vi "Test.MATLAB.vi"() -> ()   [LabVIEW 2014]
panel:
  out "Now (us)":dbl=1.0 format="%.2f"
  in  "Parameter":u16(ring) items=["Frequency (MHz)", "Amplitude (dBm)", "Phase (Pi)"]
  in  "Start":dbl=1.0 format="%.3f"
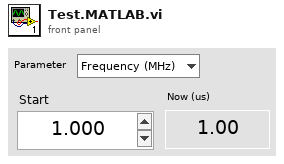
[diagram p1: front panel]
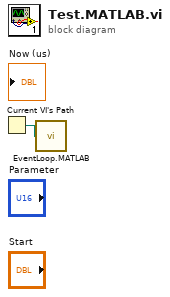
[diagram p0: block diagram]
diagram:
  n1 = Current VI's Path() -> (path=w1:path)
  n2 = call "EventLoop.MATLAB.vi"("Path"=w1) -> ()
